vi "题目3温度测量子VI.vi"() -> ()   [LabVIEW 2017]
panel:
  out "温度":string
  in  "温度单位":bool
  in  "停止":bool
  out "温度计":dbl(slide) scale=0.0..200.0
  # "℉"
  # "℃"
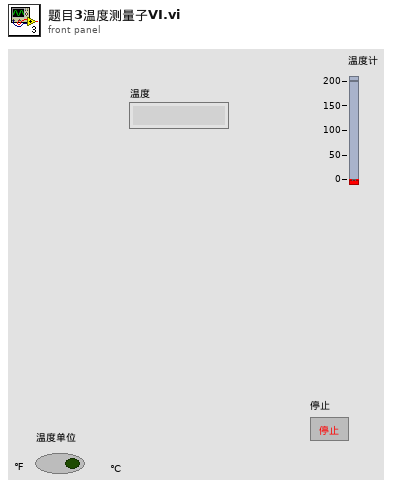
[diagram p1: front panel]
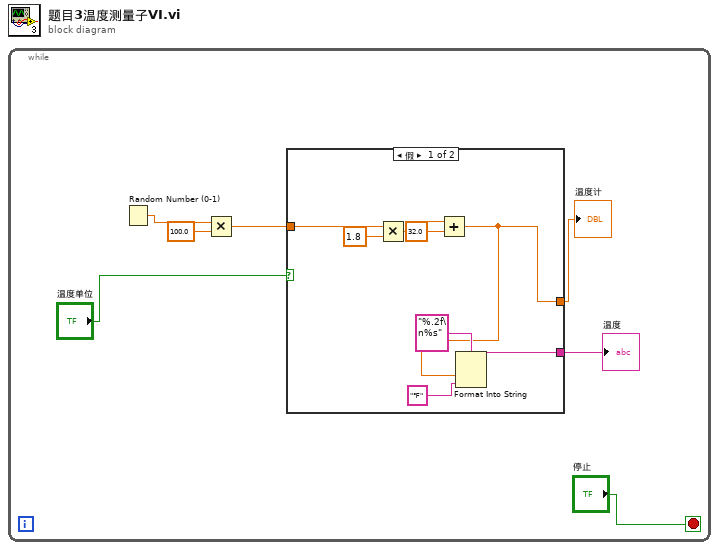
[diagram p0: block diagram]
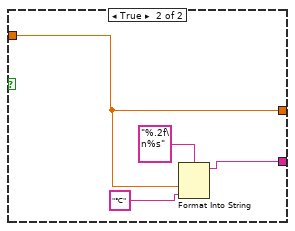
[diagram p2: hidden frame]
diagram:
  n1 = while {
    stop <- "停止" stop-if-true
    n2 = Random Number (0-1)() -> (number: 0 to 1=w7:dbl)
    n3 = Multiply(x=w7, y=100.0) -> (x*y=w4:dbl)
    n4 = case shown="假" "温度单位" {
      tunnel: [w8 w17] -> w3
      tunnel: w4 -> [w15 w17]
      tunnel: [w11 w19] -> w1
      frame False {
        n5 = Multiply(x=w15, y=1.8) -> (x*y=w13:dbl)
        n6 = Add(x=w13, y=32.0) -> (x+y=w8:dbl)
        n7 = Format Into String(format string="%.2f\n%s" ("格式字符串"), w8, "℉" ("初始字符串")) -> (resulting string=w11:string)  [unwired: 2 in, 1 out]
      }
      frame True {
        n8 = Format Into String(format string="%.2f\n%s" ("格式字符串"), w17, "℃" ("初始字符串")) -> (resulting string=w19:string)  [unwired: 2 in, 1 out]
      }
    }
    "温度计" <- w3
    "温度" <- w1
  }
